vi "Config Zero.vi"(7 "Zero Mode (off)":bool, 8 "error in":errorcluster, 9 "Loss Point (0 jpF)":dbl min=-99999999.0 max=99999999.0 format="%#_10f", 10 "Capacitance Point (0 pF)":dbl min=-99999999.0 max=99999999.0 format="%#_10f", 11 "VISA resource name":refnum<visa-resource-name>) -> (0 "error out":errorcluster, 3 "VISA resource name out":refnum<visa-resource-name>)   [LabVIEW 2017, in "Andeen-Hagerling 2700.lvlib"]
uses:
  Andeen-Hagerling 2700.lvlib
panel:
  # "Zero Parameters"
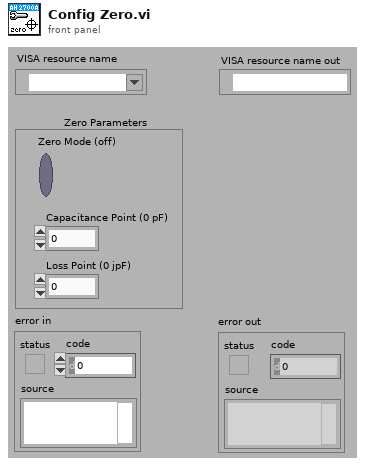
[diagram p1: front panel]
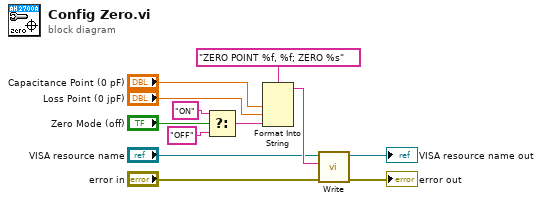
[diagram p0: block diagram]
diagram:
  n1 = Select(t="ON", s="Zero Mode (off)", f="OFF") -> (s? t:f=w2:string)
  n2 = Format Into String(format string="ZERO POINT %f, %f; ZERO %s", "Capacitance Point (0 pF)", "Loss Point (0 jpF)", w2) -> (resulting string=w10:string)  [unwired: 2 in, 1 out]
  n3 = call "Write.vi"("error in"="error in", "command"=w10, "VISA resource name"="VISA resource name") -> ("error out"=→"error out":errorcluster, "VISA resource name out"=→"VISA resource name out":refnum<visa-resource-name>)  [unwired: 7 in]
